vi "UI_Lubricate_Unit.vi"() -> ()   [LabVIEW 2014]
panel:
  out "DATA":T1
  in  "退出":bool
  # "试验单元监测参数"
  # "报警信息"
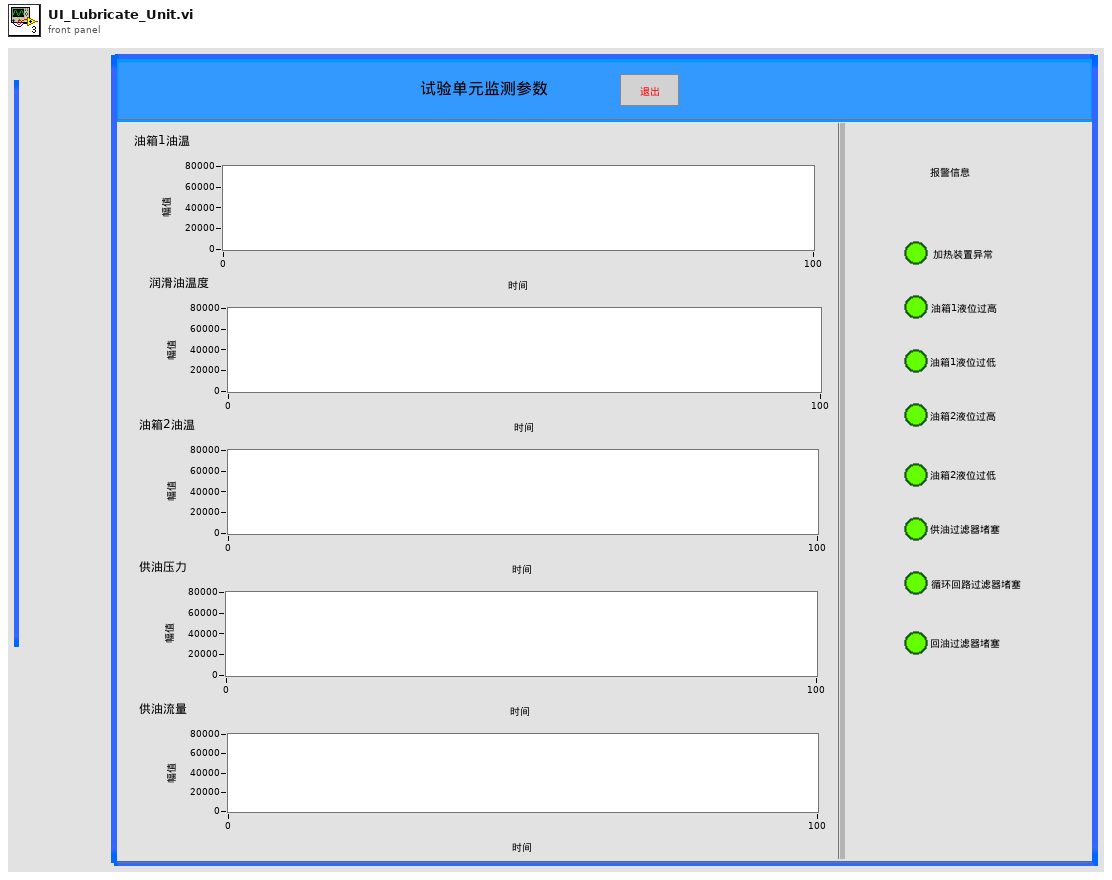
[diagram p1: front panel]
types:
  T1 = cluster{"油箱1油温 ":cluster{"油箱1油液温度":dbl, "油箱1油液温度":u16}, "润滑油温度":cluster{"润滑油温度T2最小值":dbl, "润滑油温度T2最大值":dbl, "润滑油温度":u16}, "油箱2油温":cluster{"油箱2油液温度":dbl, "油箱2油液温度":u16}, "径向液压缸加载压力 3":cluster{"供油压力最小值":dbl, "供油压力最大值":dbl, "试验轴承供油压力":u16}, "供油流量":cluster{"供油流量L1最小值":dbl, "供油流量L1最大值":dbl, "试验轴承供油流量":u16}, "报警信息":cluster{"试验轴承单元加热装置异常":bool, "试验轴承单元油箱1液位过高":bool, "试验轴承单元油箱1液位过低":bool, "试验轴承单元油箱2液位过高":bool, "试验轴承单元油箱2液位过低":bool, "试验轴承单元供油过滤器堵塞":bool, "试验轴承单元循环回路过滤器堵塞 2":bool, "试验轴承单元回油过滤器堵塞  ":bool}}
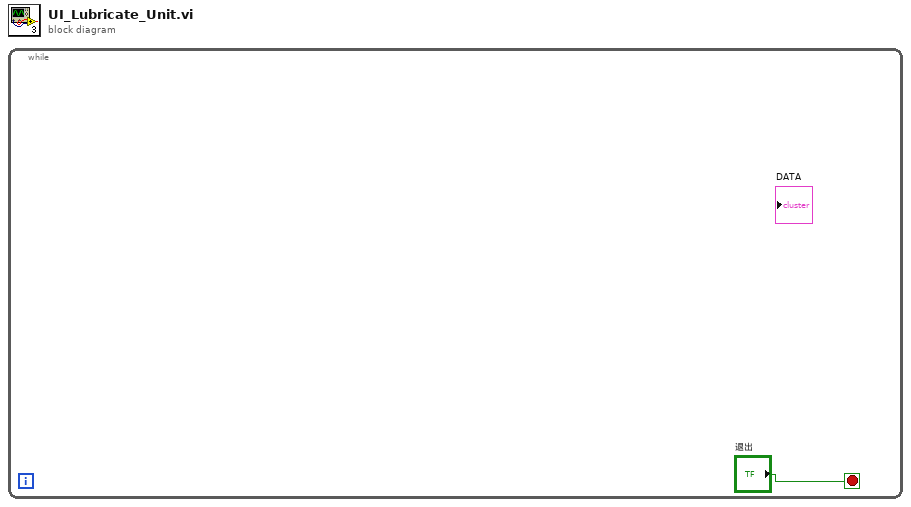
[diagram p0: block diagram]
diagram:
  n1 = while {
    stop <- "退出" stop-if-true
  }
